vi "Destroy Loader.vi"(6 "timeout (ms)":i32=5000, 8 "error in":errorcluster, 10 "Loader Name":string, 11 "gRPC ID in":T1) -> (0 "error out":errorcluster, 3 "gRPC ID out":T1)   [LabVIEW 2021, in "CIFManagerClientWrapper.lvlib"]
uses:
  CIFManagerClientWrapper.lvlib
  <vilib>/gRPC/LabVIEW gRPC Library/Shared/grpcId.ctl
  CIF_Manager_client/RPC Messages/cif_manager_DestroyPluginLoaderRequest.ctl
  CIF_Manager_client/CIF_Manager_client.lvlib
  <vilib>/gRPC/LabVIEW gRPC Library/grpc-lvsupport-release.lvlib
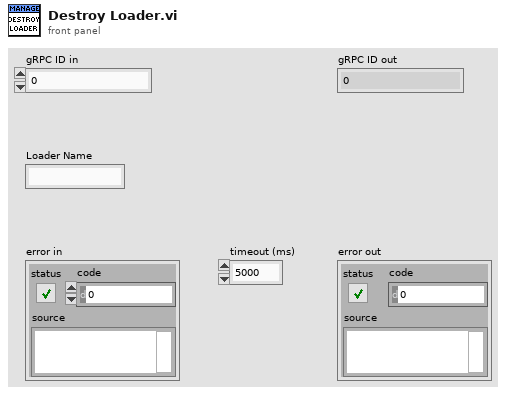
[diagram p1: front panel]
types:
  T1 = typedef "grpc-lvsupport-release.lvlib/grpcId.ctl" = u64
  T2 = typedef "CIF_Manager_client.lvlib/cif_manager_DestroyPluginLoaderRequest.ctl" = cluster{"loader_name":string}
  T3 = typedef "CIF_Manager_client.lvlib/cif_manager_DestroyPluginLoaderResponse.ctl" = cluster{"status":T4}
  T4 = typedef "CIF_Manager_client.lvlib/cif_common_Status.ctl" = cluster{"code":i32, "message":string}
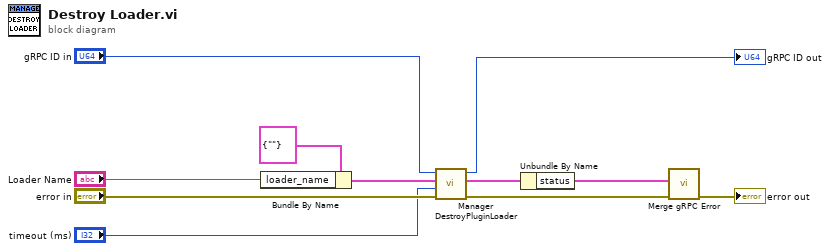
[diagram p0: block diagram]
diagram:
  n1 = Bundle By Name(cluster=T2 {"loader_name"=""} ("Request Data"), "loader_name"="Loader Name") -> (w4:T2)
  n2 = call "Manager DestroyPluginLoader.vi"("error in"="error in", "timeout (ms)"="timeout (ms)", "Request Data"=w4, "gRPC ID"="gRPC ID in") -> ("error out"=w7:errorcluster, "Response Data"=w3:T3, "gRPC ID out"=→"gRPC ID out":T1)  [unwired: 5 in]
  n3 = Unbundle By Name(w3) -> ("status"=w2:T4)
  n4 = call "Merge gRPC Error.vi"("error in (no error)"=w7, "gRPC Error"=w2) -> ("error out"=→"error out":errorcluster)  [unwired: 9 in]
